vi "Compare Version Descriptors.vi"(8 "Error In":errorcluster, 9 "Version Description 2":T1={"Major Version Number"=0, "Minor Version Number"=0, "Revision Number"=0, "Version Type"=enum."release", "a/b/rc/ Version Number"=0}, 11 "Version Description 1":T1={"Major Version Number"=0, "Minor Version Number"=0, "Revision Number"=0, "Version Type"=enum."release", "a/b/rc/ Version Number"=0}) -> (0 "Error Out":errorcluster, 2 "Version 1 = Version 2":bool, 3 "Version 1 > Version 2":bool)   [LabVIEW 2021, in "Utilities.lvlib"]
uses:
  Utilities.lvlib
  Version Description.ctl
  Version Type.ctl
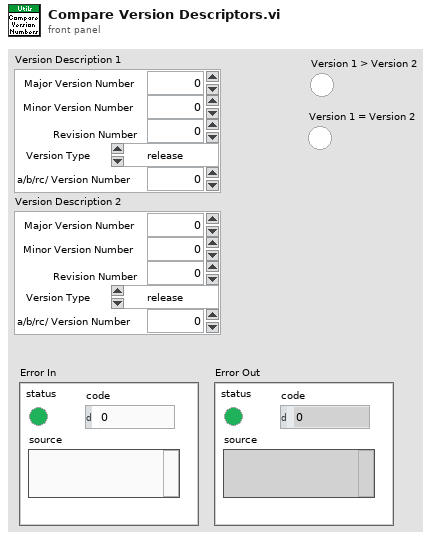
[diagram p1: front panel]
types:
  T1 = typedef "Utilities.lvlib/Version Description.ctl" = cluster{"Major Version Number":i32, "Minor Version Number":i32, "Revision Number":i32, "Version Type":T2, "a/b/rc/ Version Number":i32}
  T2 = typedef "Utilities.lvlib/Version Type.ctl" = enum16{"alpha", "beta", "release candidate", "release"}
  T3 = enum16{"major", "minor", "revision", "type", "type number"}
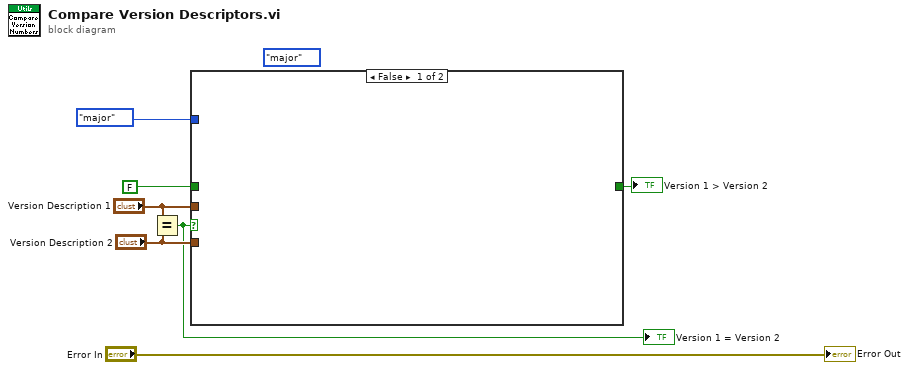
[diagram p0: block diagram]
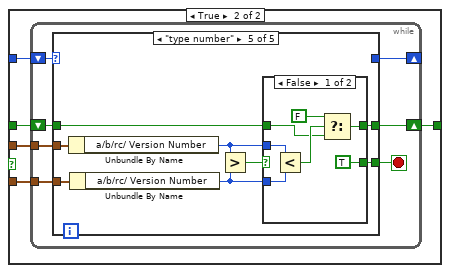
[diagram p2: hidden frame]
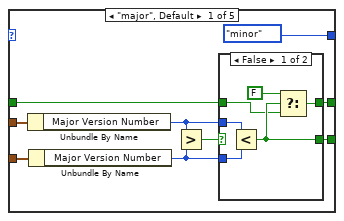
[diagram p3: hidden frame]
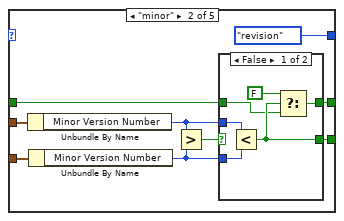
[diagram p5: hidden frame]
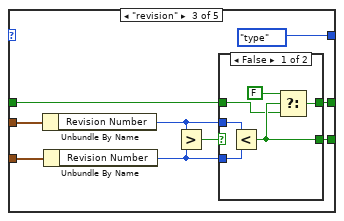
[diagram p7: hidden frame]
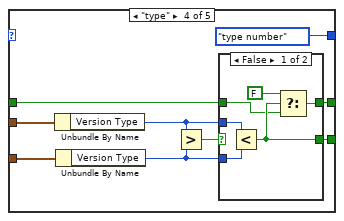
[diagram p9: hidden frame]
diagram:
  (unwired) T3."major"
  n1 = Equal?(x="Version Description 1", y="Version Description 2") -> (x = y?=w1:bool)
  "Version 1 = Version 2" <- w1
  n2 = case shown="False" w1 {
    tunnel: T3."major" -> [_ w12]
    tunnel: FALSE ("Version 1 > Version 2") -> [_ w11]
    tunnel: [_ w10] -> w4
    tunnel: "Version Description 1" -> [_ w9]
    tunnel: "Version Description 2" -> [_ w8]
    frame False {
    }
    frame True {
      n3 = while {
        tunnel: w9 -> [w19]
        tunnel: w8 -> [w18]
        shift-right: [w15] -> w10
        shift-left: w11 -> [w14]
        shift-right: [w13] -> _
        shift-left: w12 -> [w17]
        stop <- w16 stop-if-true
        n4 = case shown="\"type number\"" w17 {
          tunnel: w19 -> [w28 w44 w60 w76 w91]
          tunnel: w18 -> [w27 w43 w59 w75 w90]
          tunnel: [w25 w41 w57 w73 w88] -> w16
          tunnel: [w24 w40 w56 w72 w87] -> w15
          tunnel: w14 -> [w21 w37 w53 w69 w84]
          tunnel: [T3."minor" T3."revision" T3."type" T3."type number" _] -> w13
          frame "major", Default {
            n5 = Unbundle By Name(w28) -> ("Major Version Number"=w23:i32)
            n6 = Unbundle By Name(w27) -> ("Major Version Number"=w22:i32)
            n7 = Greater?(x=w23, y=w22) -> (0:w26:bool)
            n8 = case shown="False" w26 {
              selector: w26 -> [_ w35]
              tunnel: [w32 w35] -> w25
              tunnel: [w31 w35] -> w24
              tunnel: w23 -> [w34 _]
              tunnel: w22 -> [w33 _]
              tunnel: w21 -> [w30 _]
              frame False {
                n9 = Less?(x=w34, y=w33) -> (x < y?=w32:bool)
                n10 = Select(t=FALSE, s=w32, f=w30) -> (s? t:f=w31:bool)
              }
              frame True {
              }
            }
          }
          frame "minor" {
            n11 = Unbundle By Name(w44) -> ("Minor Version Number"=w39:i32)
            n12 = Unbundle By Name(w43) -> ("Minor Version Number"=w38:i32)
            n13 = Greater?(x=w39, y=w38) -> (0:w42:bool)
            n14 = case shown="False" w42 {
              selector: w42 -> [_ w51]
              tunnel: [w48 w51] -> w41
              tunnel: [w47 w51] -> w40
              tunnel: w39 -> [w50 _]
              tunnel: w38 -> [w49 _]
              tunnel: w37 -> [w46 _]
              frame False {
                n15 = Less?(x=w50, y=w49) -> (x < y?=w48:bool)
                n16 = Select(t=FALSE, s=w48, f=w46) -> (s? t:f=w47:bool)
              }
              frame True {
              }
            }
          }
          frame "revision" {
            n17 = Unbundle By Name(w60) -> ("Revision Number"=w55:i32)
            n18 = Unbundle By Name(w59) -> ("Revision Number"=w54:i32)
            n19 = Greater?(x=w55, y=w54) -> (0:w58:bool)
            n20 = case shown="False" w58 {
              selector: w58 -> [_ w67]
              tunnel: [w64 w67] -> w57
              tunnel: [w63 w67] -> w56
              tunnel: w55 -> [w66 _]
              tunnel: w54 -> [w65 _]
              tunnel: w53 -> [w62 _]
              frame False {
                n21 = Less?(x=w66, y=w65) -> (x < y?=w64:bool)
                n22 = Select(t=FALSE, s=w64, f=w62) -> (s? t:f=w63:bool)
              }
              frame True {
              }
            }
          }
          frame "type" {
            n23 = Unbundle By Name(w76) -> ("Version Type"=w71:T2)
            n24 = Unbundle By Name(w75) -> ("Version Type"=w70:T2)
            n25 = Greater?(x=w71, y=w70) -> (0:w74:bool)
            n26 = case shown="False" w74 {
              selector: w74 -> [_ w83]
              tunnel: [w80 w83] -> w73
              tunnel: [w79 w83] -> w72
              tunnel: w71 -> [w82 _]
              tunnel: w70 -> [w81 _]
              tunnel: w69 -> [w78 _]
              frame False {
                n27 = Less?(x=w82, y=w81) -> (x < y?=w80:bool)
                n28 = Select(t=FALSE, s=w80, f=w78) -> (s? t:f=w79:bool)
              }
              frame True {
              }
            }
          }
          frame "type number" {
            n29 = Unbundle By Name(w91) -> ("a/b/rc/ Version Number"=w86:i32)
            n30 = Unbundle By Name(w90) -> ("a/b/rc/ Version Number"=w85:i32)
            n31 = Greater?(x=w86, y=w85) -> (0:w89:bool)
            n32 = case shown="False" w89 {
              selector: w89 -> [_ w99]
              tunnel: [TRUE w99] -> w88
              tunnel: [w95 w99] -> w87
              tunnel: w86 -> [w98 _]
              tunnel: w85 -> [w97 _]
              tunnel: w84 -> [w94 _]
              frame False {
                n33 = Less?(x=w98, y=w97) -> (x < y?=w96:bool)
                n34 = Select(t=FALSE, s=w96, f=w94) -> (s? t:f=w95:bool)
              }
              frame True {
              }
            }
          }
        }
      }
    }
  }
  "Version 1 > Version 2" <- w4
  "Error Out" <- "Error In"
